vi "Format Dose Reports.vi"(0 "Volunteer ID":i32, 1 "Probability above threshold [%]":dbl=40.0, 2 "Estimated Dose Range":string, 4 "Acceptable Measurement?":bool, 5 "Main Dose Calibration Cluster":T1={"Dose Response"={"grand_mean"=0.0372961188, "slope"=0.0115712882}, "Dose Correction"={"Sex"=1, "a0"=7.719669421, "a1"=-2.746550736, "a2"=-0.186490355, "a3"=0.041922063, "a4"=-0.849147359, "a5"=0.14330063, "a6"=0.019930219, "A_n"=40.0, "H_n"=10.95, "Dose Correction"=TRUE}, "Dose Reporting"={"Reporting is"=TRUE, "sd_threshold [AU]"=0.06, "sd_model [Gy]"=0.66, "dosimetric_threshold [Gy]"=2.0, "Add intrasession errors is"=TRUE, "Prior Radiation?"=TRUE}} {"Dose Reporting"."dosimetric_threshold [Gy]" format="%#_9g"; "Dose Reporting"."sd_model [Gy]" format="%#_9g"; "Dose Reporting"."sd_threshold [AU]" format="%#_9g"; "Dose Correction"."H_n" format="%#_9g"; "Dose Correction"."A_n" format="%#_9g"; "Dose Correction"."a6" format="%#.9g"; "Dose Correction"."a5" format="%#.9g"; "Dose Correction"."a4" format="%#.9g"; "Dose Correction"."a3" format="%#.9g"; "Dose Correction"."a2" format="%#.9g"; "Dose Correction"."a1" format="%#.9g"; "Dose Correction"."a0" format="%#.9g"; "Dose Correction"."Sex" items=["Male"=1, "Female"=0]; "Dose Response"."slope" format="%#_9g"; "Dose Response"."grand_mean" format="%#_9g"}) -> (17 "Reporting String":string)   [LabVIEW 2016]
uses:
  Dose Calculation Control.ctl
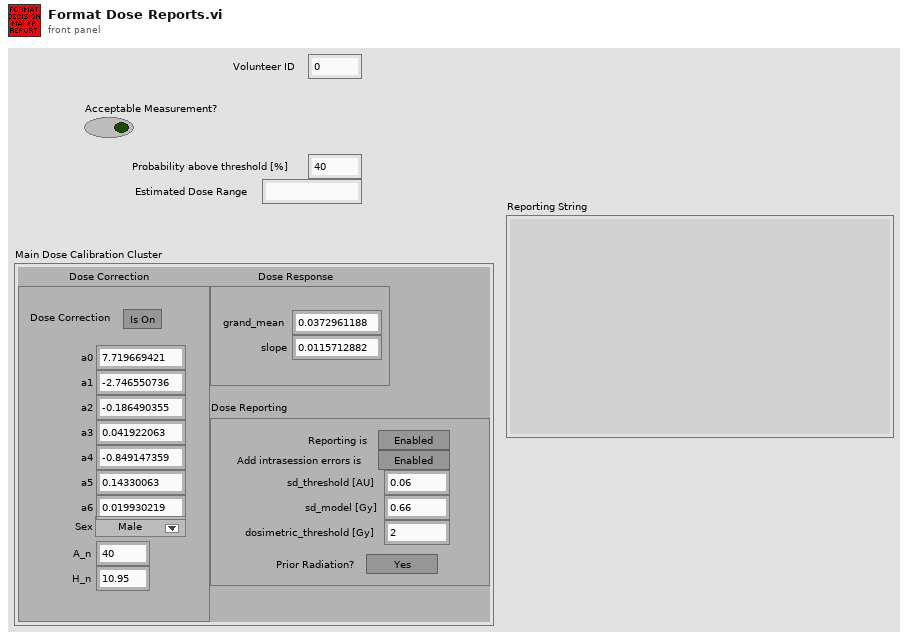
[diagram p1: front panel]
types:
  T1 = typedef "Dose Calculation Control.ctl" = cluster{"Dose Response":cluster{"grand_mean":dbl, "slope":dbl}, "Dose Correction":cluster{"Sex":u16, "a0":dbl, "a1":dbl, "a2":dbl, "a3":dbl, "a4":dbl, "a5":dbl, "a6":dbl, "A_n":dbl, "H_n":dbl, "Dose Correction":bool}, "Dose Reporting":cluster{"Reporting is":bool, "sd_threshold [AU]":dbl, "sd_model [Gy]":dbl, "dosimetric_threshold [Gy]":dbl, "Add intrasession errors is":bool, "Prior Radiation?":bool}}
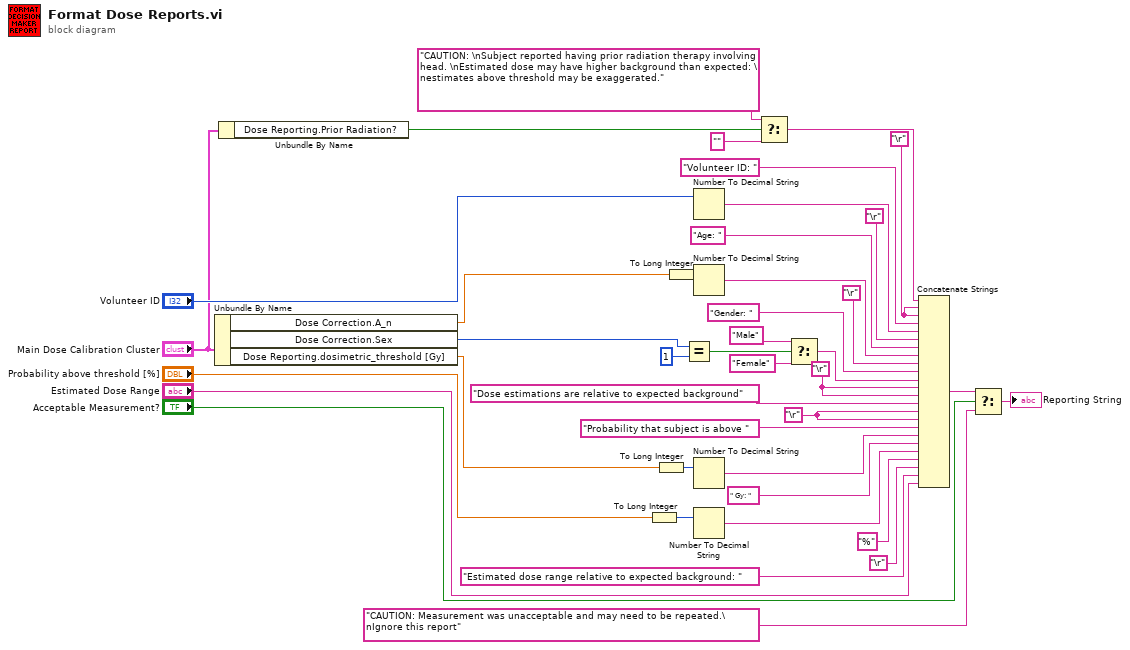
[diagram p0: block diagram]
diagram:
  w8 = "\r"
  w22 = "\r"
  w24 = "\r"
  n1 = Unbundle By Name("Main Dose Calibration Cluster") -> ("Dose Correction.A_n"=w11:dbl, "Dose Correction.Sex"=w10:u16, "Dose Reporting.dosimetric_threshold [Gy]"=w9:dbl)
  n2 = Unbundle By Name("Main Dose Calibration Cluster") -> ("Dose Reporting.Prior Radiation?"=w2:bool)
  n3 = To Long Integer(number="Probability above threshold [%]") -> (32bit integer=w26:i32)
  n4 = To Long Integer(number=w9) -> (32bit integer=w28:i32)
  n5 = To Long Integer(number=w11) -> (32bit integer=w29:i32)
  n6 = Equal?(x=w10, y=u16 1) -> (x = y?=w37:bool)
  n7 = Number To Decimal String(number="Volunteer ID") -> (decimal integer string=w35:string)  [unwired: 1 in]
  n8 = Number To Decimal String(number=w29) -> (decimal integer string=w40:string)  [unwired: 1 in]
  n9 = Number To Decimal String(number=w28) -> (decimal integer string=w20:string)  [unwired: 1 in]
  n10 = Number To Decimal String(number=w26) -> (decimal integer string=w18:string)  [unwired: 1 in]
  n11 = Select(t="CAUTION: \nSubject reported having prior radiation therapy involving head. \nEstimated dose may have higher background than expected: \nestimates above threshold may be exaggerated." ("string"), s=w2, f="") -> (s? t:f=w7:string)
  n12 = Select(t="Male" ("string"), s=w37, f="Female" ("string")) -> (s? t:f=w31:string)
  n13 = Concatenate Strings(w7, w8, w8, "Volunteer ID: " ("string"), w35, "\r", "Age: " ("string"), w40, "\r", "Gender: " ("string"), w31, w24, w24, "Dose estimations are relative to expected background" ("string"), w22, w22, "Probability that subject is above " ("string"), w20, " Gy: " ("string"), w18, "%" ("string"), "\r", "Estimated dose range relative to expected background: " ("string"), "Estimated Dose Range") -> (w6:string)
  n14 = Select(t=w6, s="Acceptable Measurement?", f="CAUTION: Measurement was unacceptable and may need to be repeated.\nIgnore this report") -> (s? t:f=→"Reporting String":string)
